vi "Write all.vi"(7 "horizontal":bool, 8 "error in (no error)":errorcluster, 9 "Endpunkt":dbl[](array[numeric]), 10 "Startpunkt":dbl[](array[numeric]), 11 "Gerade in":refnum<class "Gerade.lvclass">) -> (0 "error out":errorcluster, 3 "Gerade out":refnum<class "Gerade.lvclass">)   [LabVIEW 2019, in "Gerade.lvclass"]
uses:
  Gerade.lvclass
  Gerade.lvclass/Gerade.ctl
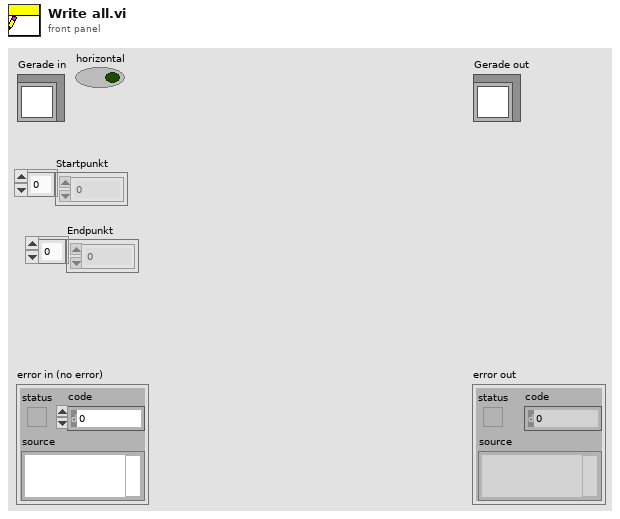
[diagram p1: front panel]
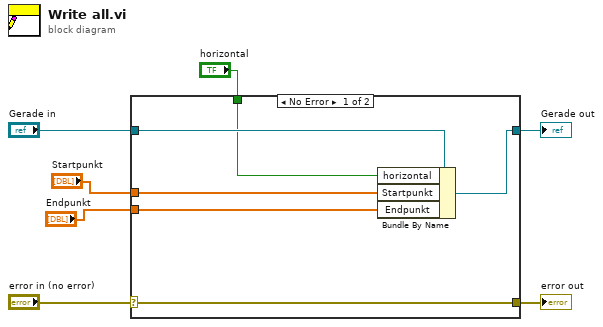
[diagram p0: block diagram]
diagram:
  n1 = case shown="No Error" "error in (no error)" {
    selector: "error in (no error)" -> [w13 w14]
    tunnel: [w13 w14] -> w6
    tunnel: [w12 w15] -> w4
    tunnel: "Gerade in" -> [w11 w15]
    tunnel: "Endpunkt" -> [w10 _]
    tunnel: "Startpunkt" -> [w9 _]
    tunnel: "horizontal" -> [w8 _]
    frame No Error {
      n2 = Bundle By Name(cluster=w11, "horizontal"=w8, "Startpunkt"=w9, "Endpunkt"=w10) -> (w12:refnum<class "Gerade.lvclass">)
    }
    frame Error {
    }
  }
  "error out" <- w6
  "Gerade out" <- w4
